vi "Marshal.vi"(8 "error in (no error)":errorcluster, 11 "Message in":refnum<class "Raw Message.lvclass">) -> (0 "error out":errorcluster, 2 "Buffer":u8[](array[numeric]), 3 "Message out":refnum<class "Raw Message.lvclass">)   [LabVIEW 2020, in "Protobuf RAW.lvlib" / "Raw Message.lvclass"]
uses:
  Raw Message.lvclass
  Raw Message.lvclass/Raw Message.ctl
  552cc200-1725-44b6-b581-55001ee92a8a.vi
  d8077f1f-2bc6-4b8d-a51a-6e66fe0f2243.vi
  552cc200-1725-44b6-b581-55001ee92a8a.vi/0f065a35-b637-42bd-ae45-04c3465bdb97.vi
  d8077f1f-2bc6-4b8d-a51a-6e66fe0f2243.vi/0f065a35-b637-42bd-ae45-04c3465bdb97.vi
  Tag/Basic Type.lvclass
  Protobuf RAW.lvlib
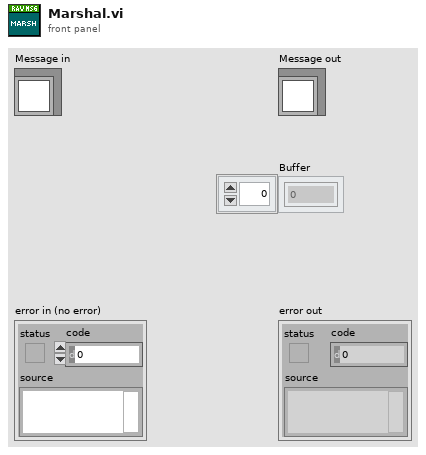
[diagram p1: front panel]
types:
  T1 = typedef "Protobuf RAW.lvlib/Wire Type Group.lvclass/Wire Type.ctl" = enum16{"VARINT", "I64", "LEN", "SGROUP", "EGROUP", "I32"}
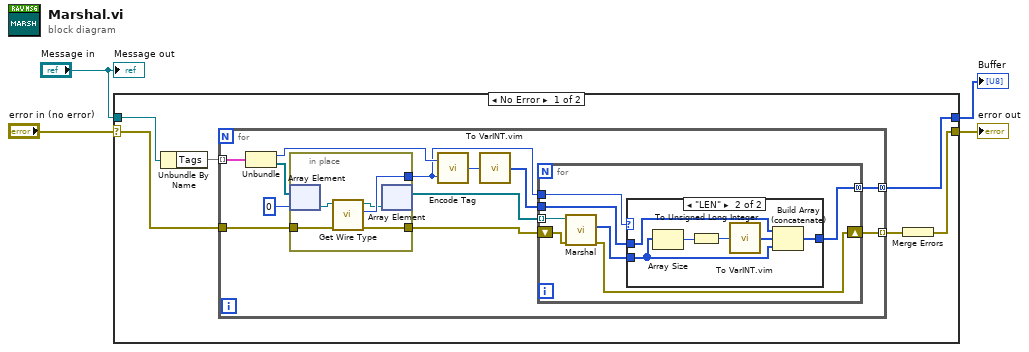
[diagram p0: block diagram]
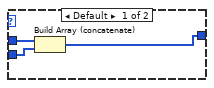
[diagram p2: hidden frame]
diagram:
  n1 = case shown="No Error" "error in (no error)" {
    selector: "error in (no error)" -> [w8 w44]
    tunnel: "Message in" -> [w10 _]
    tunnel: [w7 _] -> w2
    tunnel: [w5 w44] -> w1
    frame No Error {
      n2 = Unbundle By Name(w10) -> ("Tags"=w9:map{u32, refnum<class "Basic Type.lvclass">[]})
      n3 = for {
        tunnel: w9 -> [w22] mode=indexing
        tunnel: w8 -> [w14]
        tunnel: [w21] -> w6 mode=indexing
        tunnel: [w19] -> w7 mode=concatenating
        n4 = Unbundle(w22) -> ("ID"=w20:u32, "Tag"=w16:refnum<class "Basic Type.lvclass">[])
        n5 = in-place {
          in-place-border: w14 -> [w27]
          in-place-border: [w26] -> w13
          in-place-border: [w23] -> w11
          n6 = in-place-array #1(w16, 0) -> (w25:refnum<class "Basic Type.lvclass">)
          n7 = call-dynamic "Get Wire Type.vi"("error in (no error)"=w27, "Tag.lvclass"=w25) -> ("error out"=w23:errorcluster, "Wire Type"=w26:T1, "Tag.lvclass 2"=w24:refnum<class "Basic Type.lvclass">)  [unwired: 7 in]
          n8 = in-place-array #1(w24) -> (w15:refnum<class "Basic Type.lvclass">[])  [unwired: 1 out]
        }
        n9 = call "Encode Tag.vi"("Wire Type"=w13, "ID"=w20) -> ("Tag"=w18:u32)
        n10 = call "To VarINT.vim"("Integer"=w18) -> ("LEB128"=w17:u8[])
        n11 = for {
          tunnel: [w31] -> w19 mode=concatenating
          tunnel: w17 -> [w30]
          tunnel: w13 -> [w29]
          shift-right: [w34] -> w21
          shift-left: w11 -> [w32]
          tunnel: w15 -> [w28] mode=indexing
          n12 = call-dynamic "Marshal.vi"("error in (no error)"=w32, "Tag in"=w28) -> ("error out"=w34:errorcluster, "Buffer"=w33:u8[])  [unwired: 7 in, 1 out]
          n13 = case shown="\"LEN\"" w29 {
            tunnel: w33 -> [w37 w41]
            tunnel: [w36 w43] -> w31
            tunnel: w30 -> [w35 w42]
            frame Default {
              n14 = Build Array (concatenate)(w35, w37) -> (w36:u8[])
            }
            frame "LEN" {
              n15 = Array Size(array=w41) -> (size(s)=w40:i32)
              n16 = To Unsigned Long Integer(number=w40) -> (unsigned 32bit integer=w39:u32)
              n17 = call "To VarINT.vim"("Integer"=w39) -> ("LEB128"=w38:u8[])
              n18 = Build Array (concatenate)(w42, w38, w41) -> (w43:u8[])
            }
          }
        }
      }
      n19 = Merge Errors(w6) -> (w5:errorcluster)
    }
    frame Error {
    }
  }
  "error out" <- w1
  "Buffer" <- w2
  "Message out" <- "Message in"
